vi "SC handler interface.vi"() -> ()   [LabVIEW 2011]
doc: "This VI demonstrates how to set up a GPIB board as a non system controller to simulate an instrument using the following steps:\n\nOpen a VISA session to the GPIB interface, set it as the non-system controller, and assign it a primary address. \nUse the VISA Enable Event VI to register the \"GPIB Listener\" Event; this event occurs when the GPIB interface is addressed as a listener. \nUse the VISA Wait on Event VI to wait until the GPIB interface is a listener; this means that there is data available on the bus for the interface.\nUse the VISA Read VI to read the available data, parse it, and send an appropriate response.\nCall the VISA close VI after the stop button is pressed\n\nNote: For a description of other available VISA event types, see the NI-VISA help."
uses:
  SC virtual tester states.ctl
panel:
  out "wt end hidden":u32
  out "wt start hidden":u32
  in  "sites ready hidden":string
  out "VISA close error":bool
  out "VISA error out":errorcluster
  out "VISA resource name out":refnum<visa-resource-name>
  out "VISA open error":bool
  in  "SC virtual tester states":T1
  out "H1 active":bool
  out "H2 active":bool
  out "GPIB read error":bool
  out "GPIB write error":bool
  in  "START TEST":bool
  in  "Yield variation":dbl min=-50.0 max=0.0 step=1.0
  in  "Yield set":dbl=100.0 min=0.0 max=100.0 step=1.0
  out "Wait time":dbl format="%.2f"
  in  "Test time variation":dbl=1.0 min=0.1 max=10.0 step=0.1 format="%.2f"
  out "binning string hidden":string
  out "Test time":dbl format="%.2f"
  in  "Reset Yield":bool
  out "Waiting":bool
  out "Testing":bool
  out "Duty cycle":u32(knob) caption="Duty Cycle" scale=0.0..100.0 scale format="%#.0f"
  out "Good Devices":u64
  out "Devices Tested":u64
  out "Yield":dbl format="%#.0f"
  in  "Tester talks to Sentinel Controller at":refnum<visa-resource-name>="GPIB0::1::INSTR"
  in  "Power on/off":bool=TRUE
  in  "Parallelism set":u8=8 min=1 step=1
  out "Message from tester to Sentinel Controller":string
  out "Reply from Sentinel Controller to tester":string="Response here\n"
  out "Parallelism reported by handler":u8
  out "Parallelism mismatch":bool
  in  "Test time set":dbl=1.0 min=0.1 max=10.0 step=0.1 format="%.2f"
  # "Celerint Sentinel Controller ~ Tester Simulator"
  # "%"
  # "%"
  # "%"
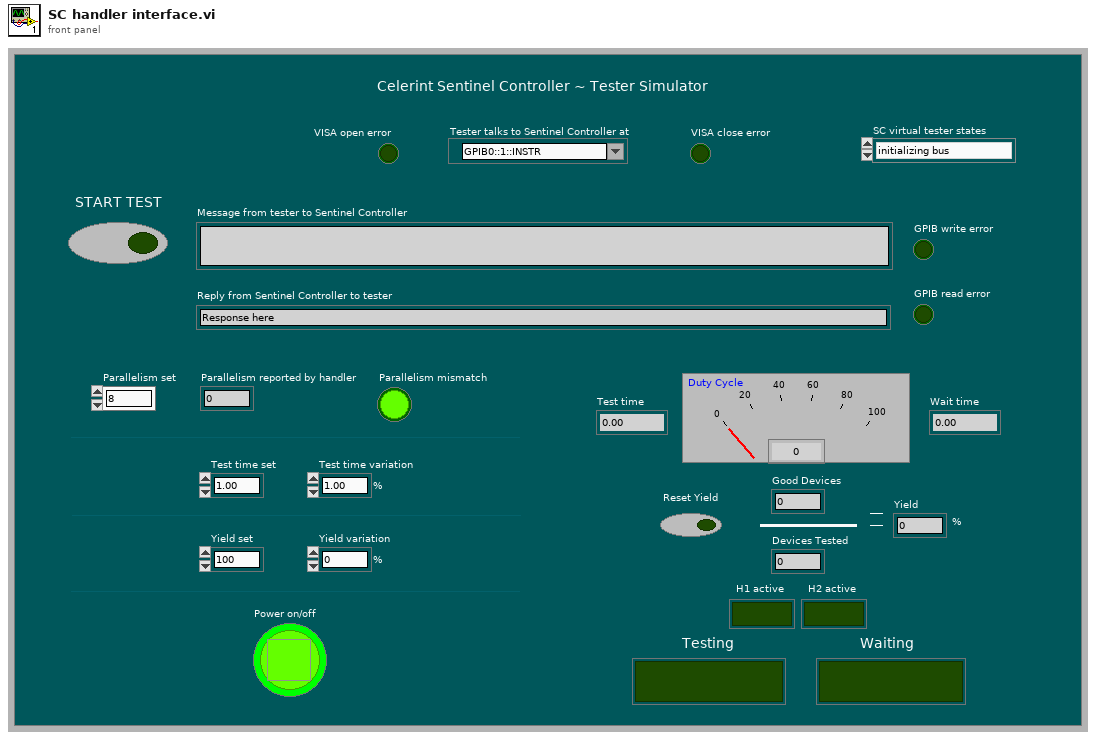
[diagram p1: front panel]
types:
  T1 = typedef "SC virtual tester states.ctl" = enum16{"initializing bus", "polling *SITES?", "sending *IDN?", "sending *HAND?", "testing", "binning", "closing bus"}
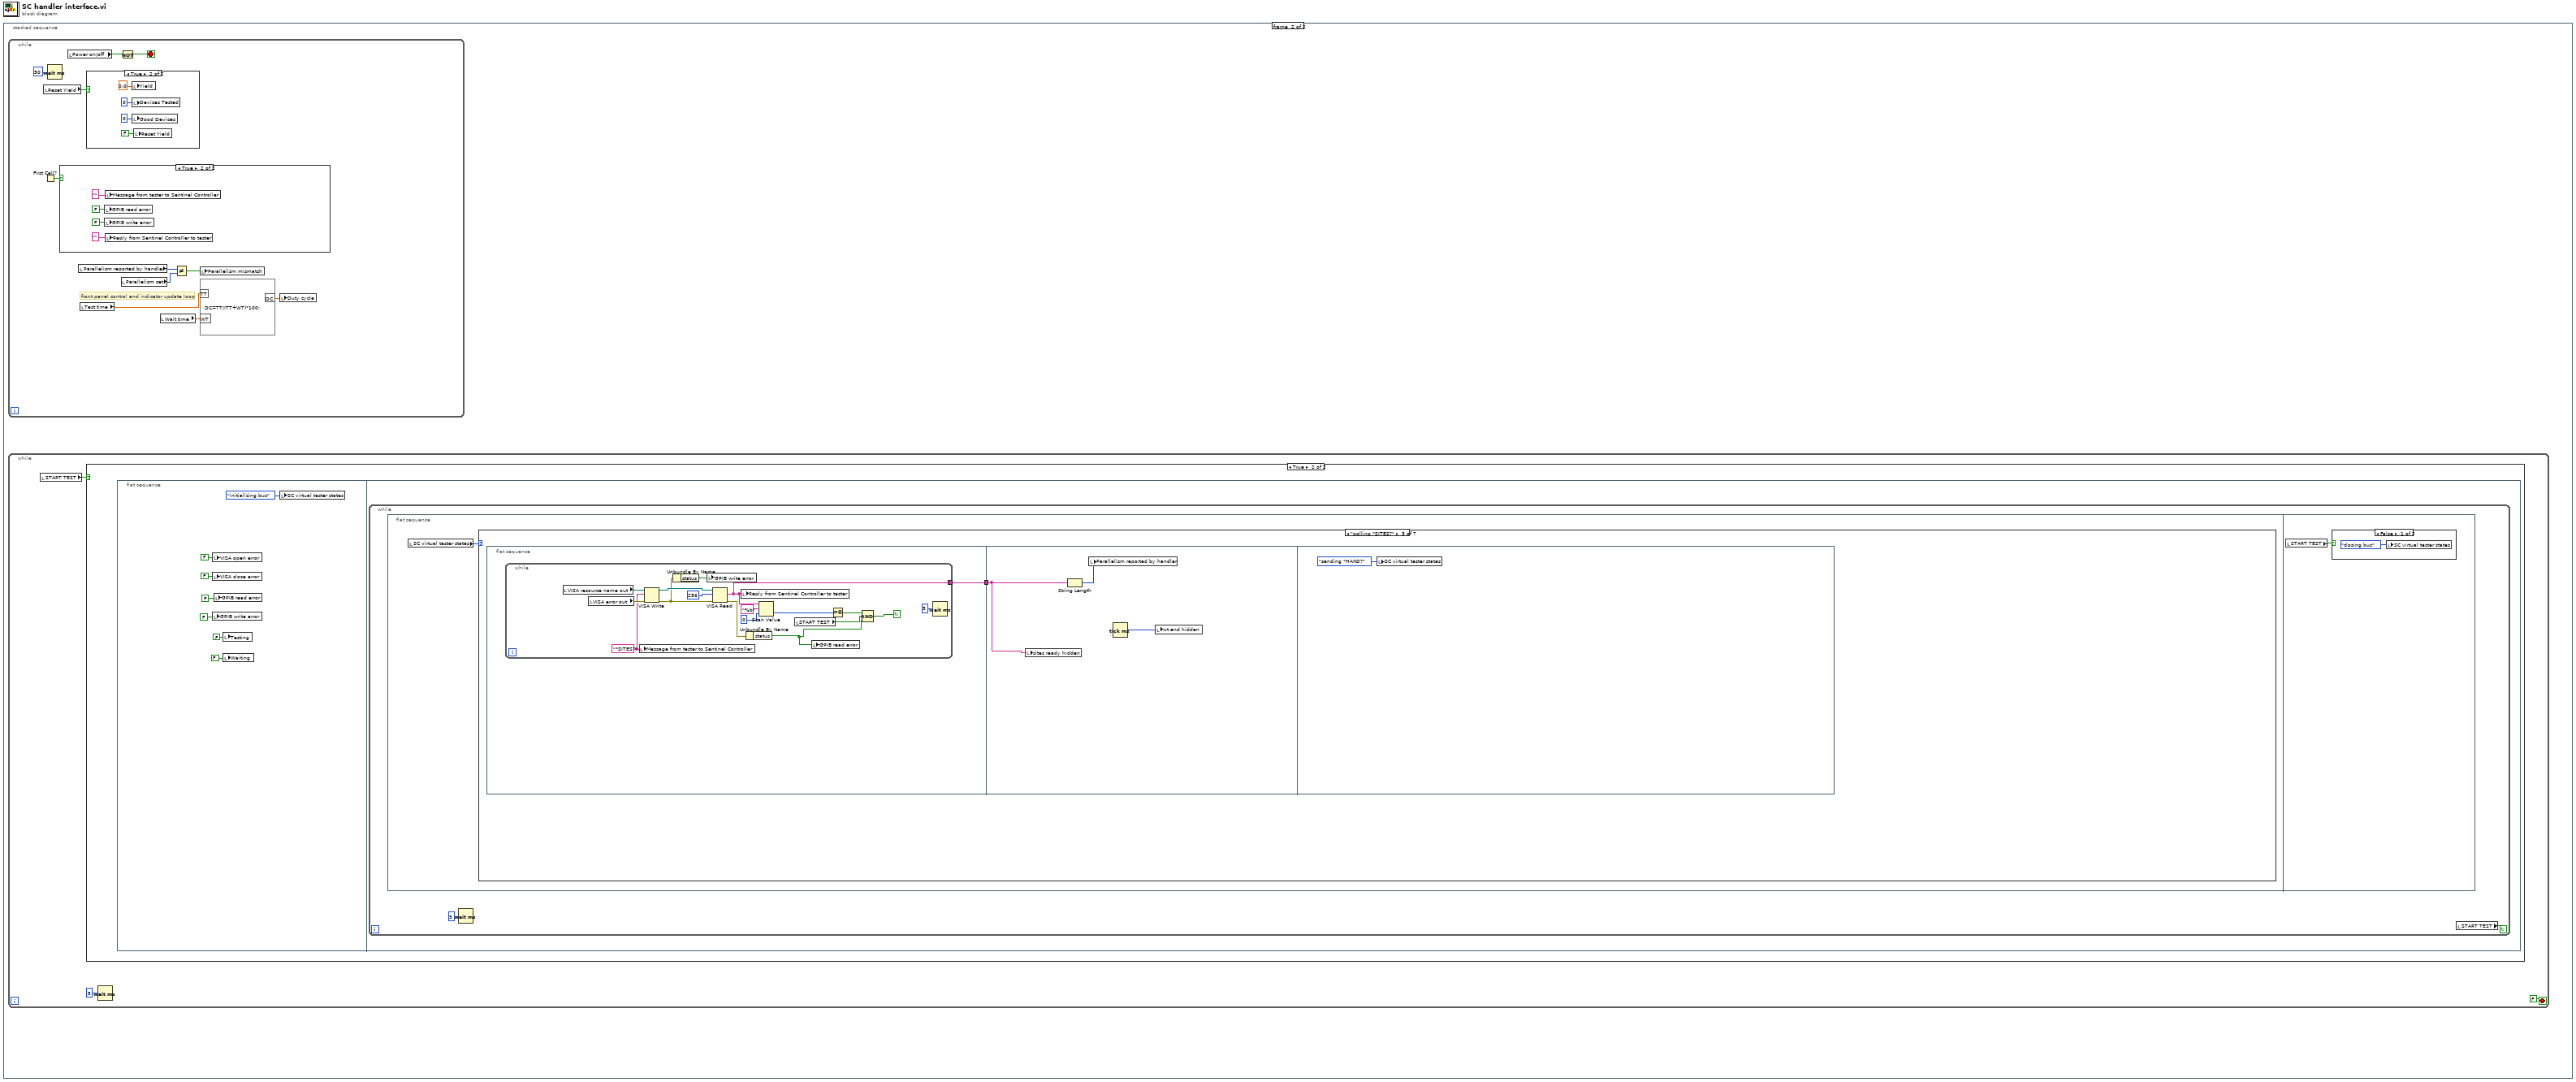
[diagram p0: block diagram]
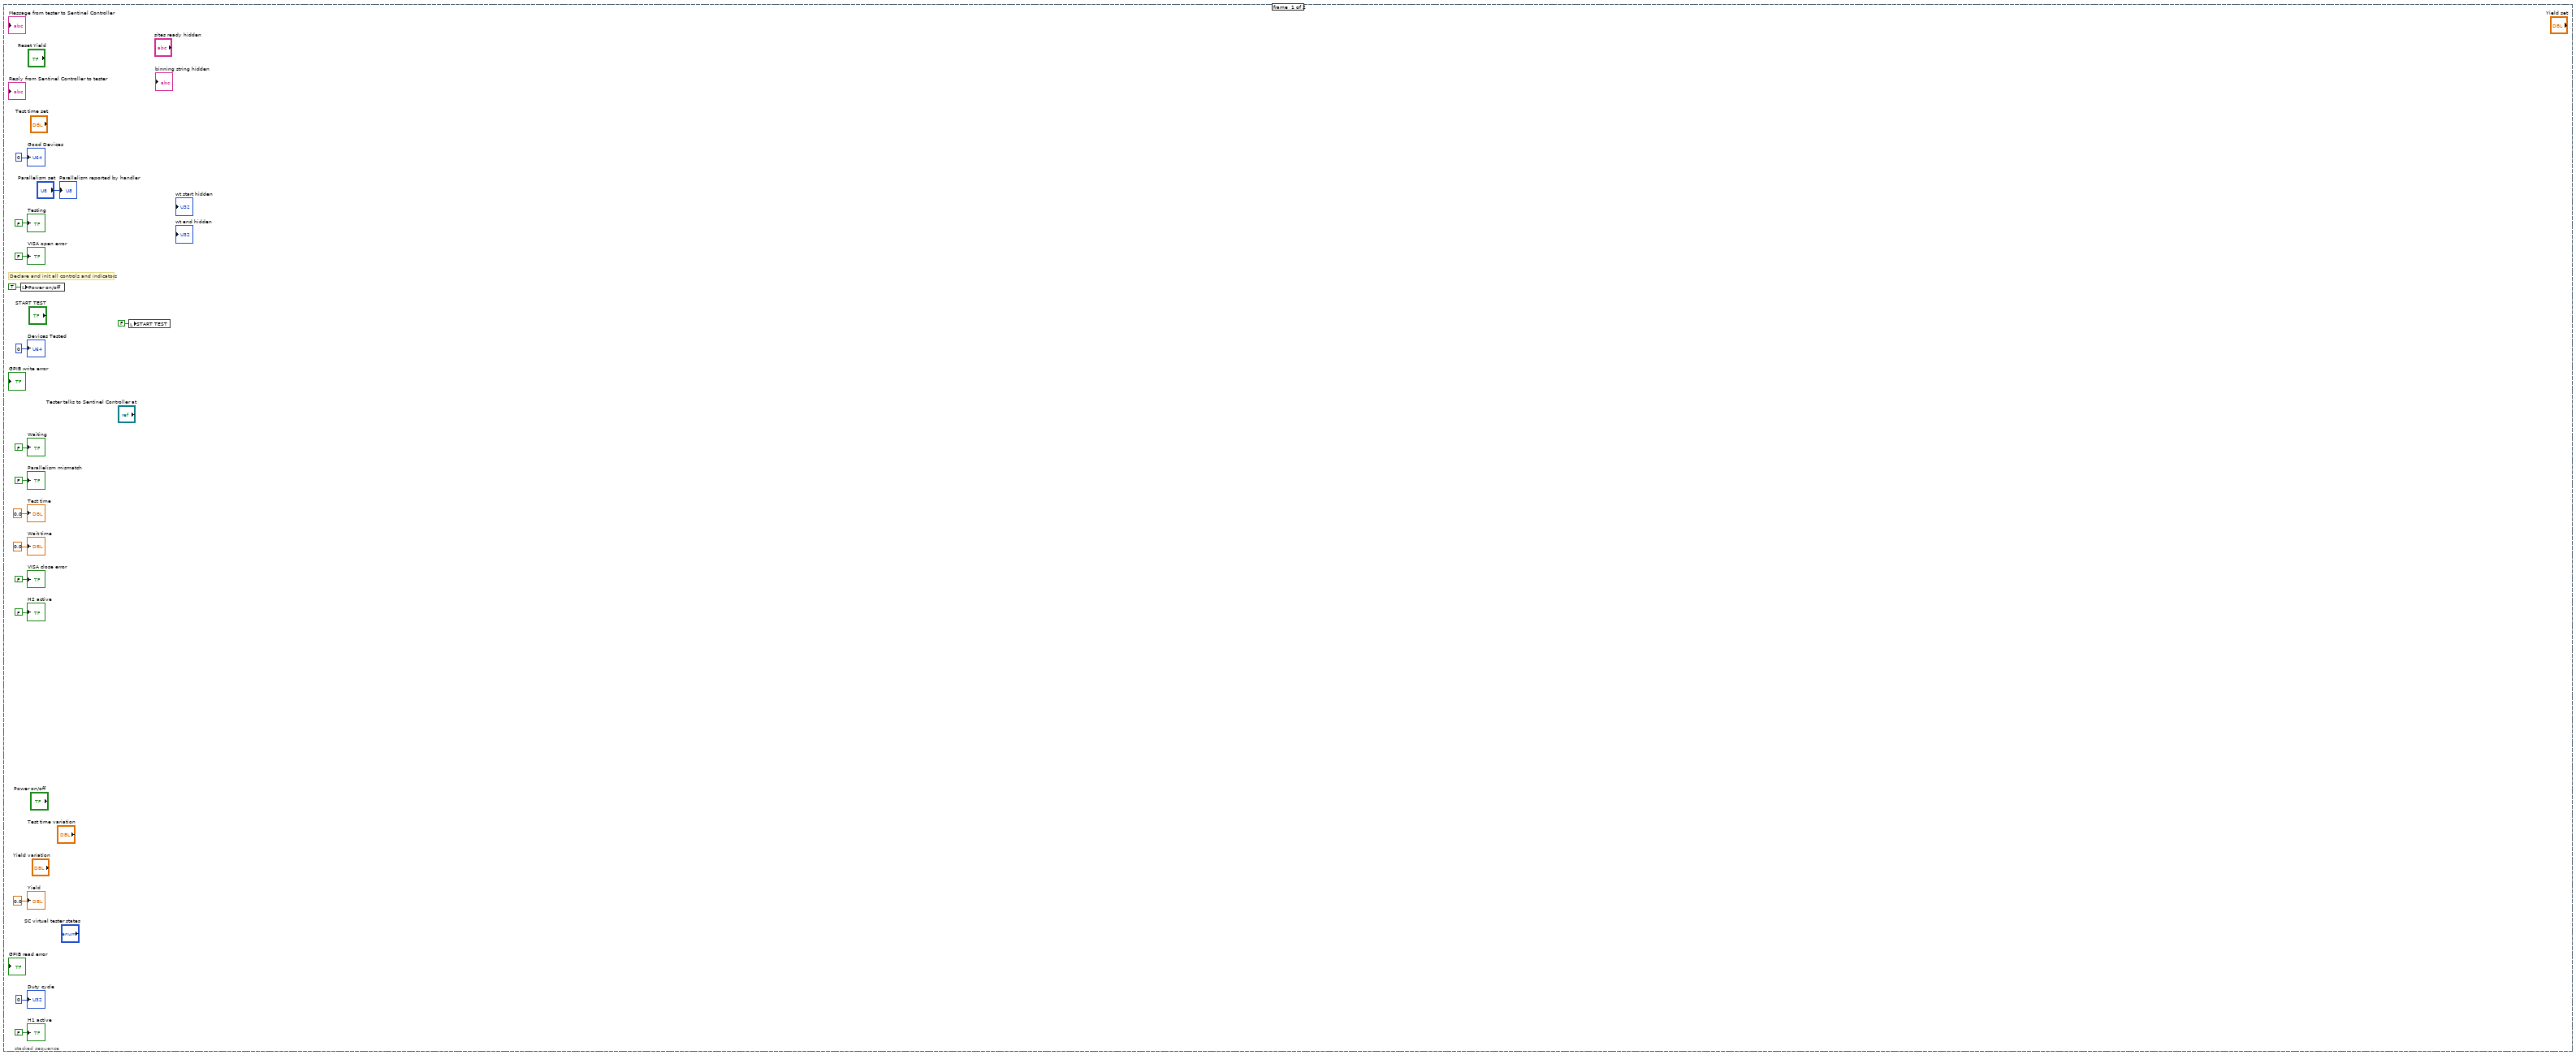
[diagram p2: hidden frame]
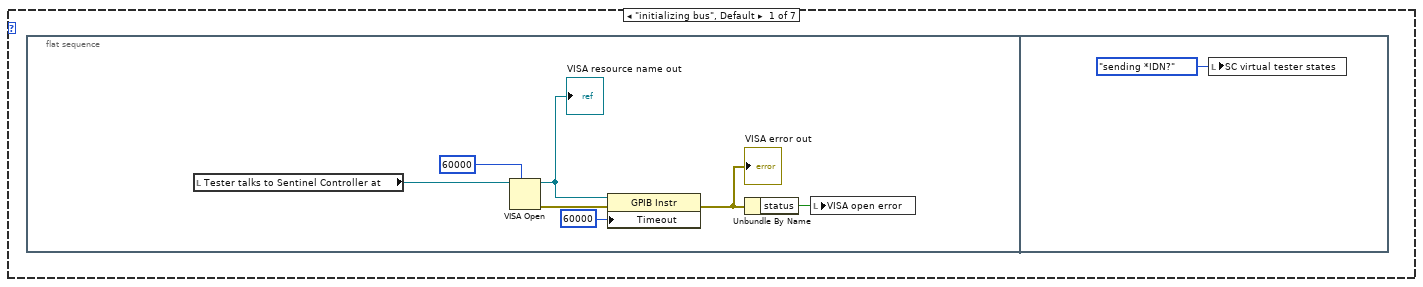
[diagram p4: hidden frame]
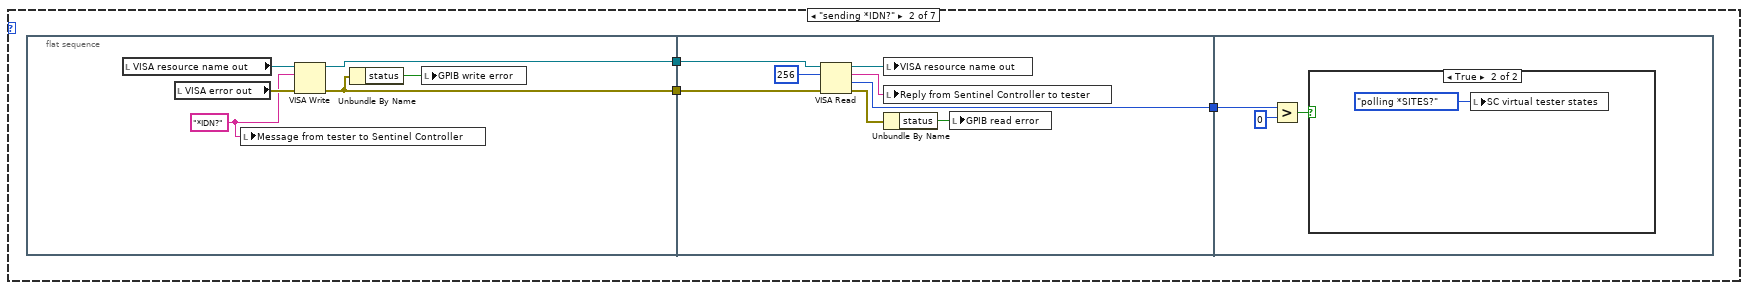
[diagram p5: hidden frame]
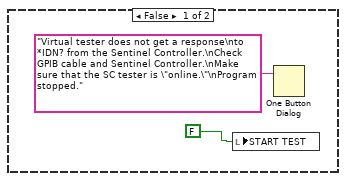
[diagram p6: hidden frame]
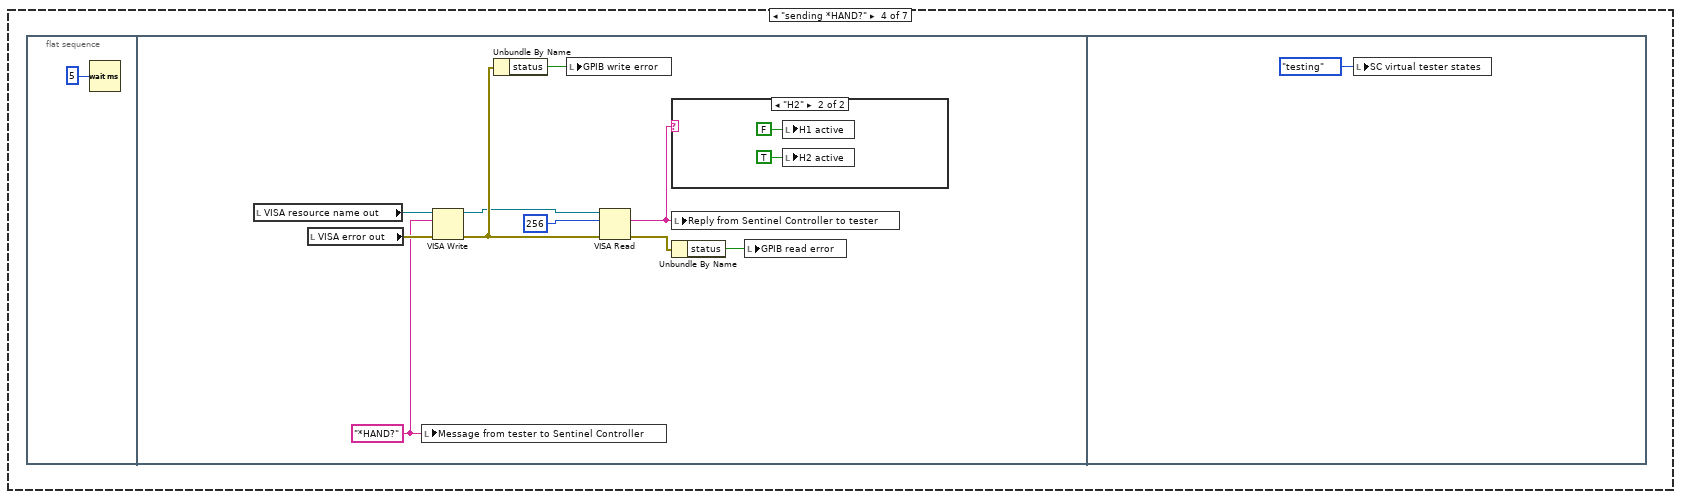
[diagram p7: hidden frame]
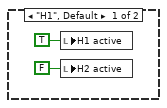
[diagram p8: hidden frame]
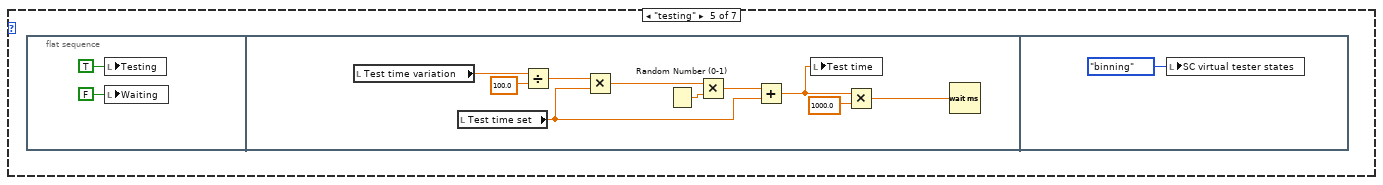
[diagram p9: hidden frame]
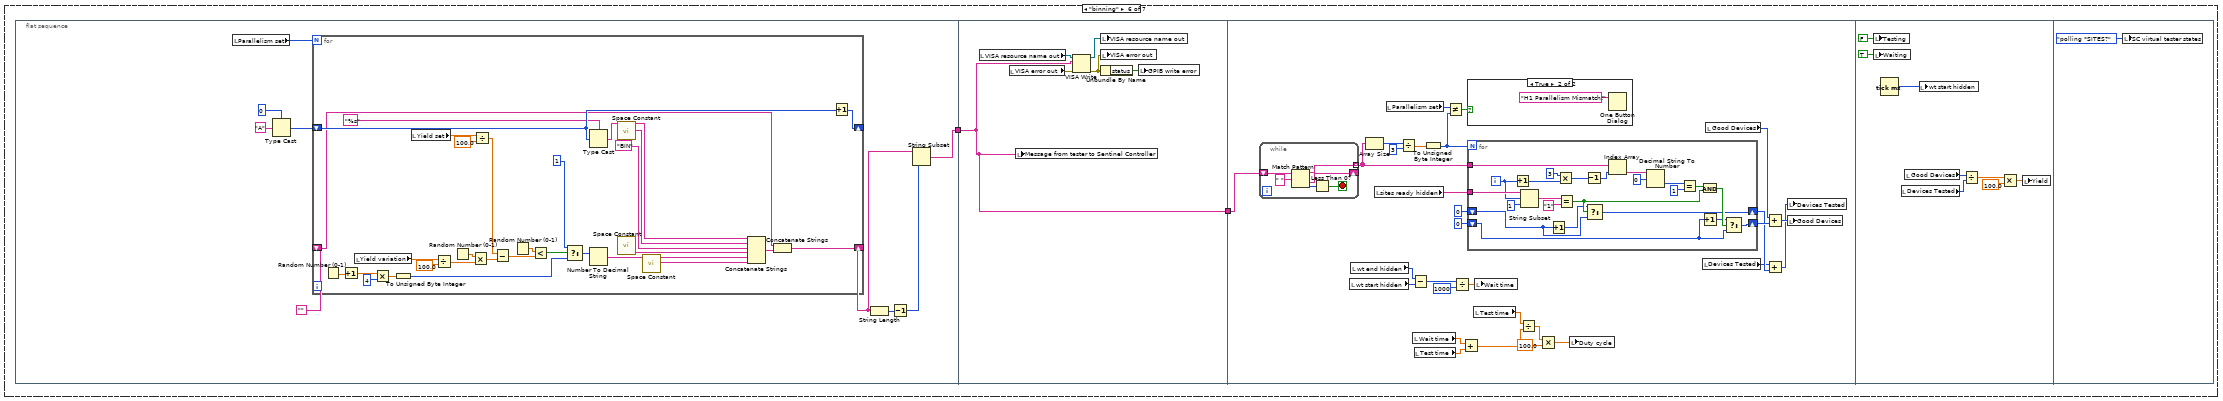
[diagram p10: hidden frame]
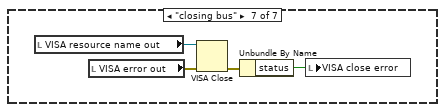
[diagram p12: hidden frame]
diagram:
  n1 = stacked-sequence {
    frame #0 {
      # "Declare and init all controls and indicators"
      n2 = local write "Power on/off"(TRUE ("Power on/off")) -> ()
      n3 = local write "START TEST"(FALSE ("START TEST")) -> ()
      "Good Devices" <- u64 0 ("Good Devices")
      "Devices Tested" <- u64 0 ("Devices Tested")
      "Yield" <- 0.0 ("Yield")
      "Waiting" <- FALSE ("Indexing")
      "Testing" <- FALSE ("Testing")
      "Duty cycle" <- u32 0 ("H1 UPH")
      "Parallelism reported by handler" <- "Parallelism set"
      "Parallelism mismatch" <- FALSE ("Parallelism mismatch")
      "Test time" <- 0.0 ("Test Time")
      "Wait time" <- 0.0 ("Wait time")
      "VISA close error" <- FALSE ("VISA close error")
      "VISA open error" <- FALSE ("VISA open error")
      "H1 active" <- FALSE ("H1 active")
      "H2 active" <- FALSE ("H2 active")
    }
    frame #1 {
      n4 = while {
        stop <- w244 stop-if-true
        # "front panel control and indicator update loop"
        n5 = local read "Reset Yield"() -> (w241:bool)
        n6 = First Call?() -> (First Call?: T/F=w237:bool)
        n7 = Wait (ms)(milliseconds to wait=u32 50) -> ()  [unwired: 1 out]
        n8 = case shown="True" w237 {
          frame False {
          }
          frame True {
            n9 = local write "GPIB read error"(FALSE ("GPIB read error")) -> ()
            n10 = local write "GPIB write error"(FALSE ("GPIB write error")) -> ()
            n11 = local write "Message from tester to Sentinel Controller"("" ("Message from tester to Sentinel Controller")) -> ()
            n12 = local write "Reply from Sentinel Controller to tester"("" ("Reply from Sentinel Controller to tester")) -> ()
          }
        }
        n13 = local read "Power on/off"() -> (w243:bool)
        n14 = local read "Parallelism reported by handler"() -> (w234:u8)
        n15 = local read "Test time"() -> (w239:dbl)
        n16 = case shown="True" w241 {
          frame False {
          }
          frame True {
            n17 = local write "Yield"(0.0 ("Yield")) -> ()
            n18 = local write "Devices Tested"(u64 0 ("Devices Tested")) -> ()
            n19 = local write "Good Devices"(u64 0 ("Good Devices")) -> ()
            n20 = local write "Reset Yield"(FALSE ("Reset Yield")) -> ()
          }
        }
        n21 = Not(x=w243) -> (.not. x?=w244:bool)
        n22 = local read "Parallelism set"() -> (w236:u8)
        n23 = local read "Wait time"() -> (w240:dbl)
        n24 = Not Equal?(x=w234, y=w236) -> (x != y?=w235:bool)
        n25 = local write "Parallelism mismatch"(w235) -> ()
        n26 = formula code="DC=TT/(TT+WT)*100;"("TT"=w239, "WT"=w240) -> ("DC"=w238:dbl)
        n27 = local write "Duty cycle"(w238) -> ()
      }
      n28 = while {
        stop <- FALSE stop-if-true
        n29 = local read "START TEST"() -> (w18:bool)
        n30 = case shown="True" w18 {
          frame False {
          }
          frame True {
            n31 = flat-sequence {
              frame #0 {
                n32 = local write "VISA open error"(FALSE ("VISA open error")) -> ()
                n33 = local write "VISA close error"(FALSE ("VISA open error")) -> ()
                n34 = local write "GPIB write error"(FALSE ("VISA open error")) -> ()
                n35 = local write "GPIB read error"(FALSE ("VISA open error")) -> ()
                n36 = local write "Testing"(FALSE ("VISA open error")) -> ()
                n37 = local write "Waiting"(FALSE ("VISA open error")) -> ()
                n38 = local write "SC virtual tester states"(SC_virtual_tester_states."initializing bus" ("SC virtual tester states")) -> ()
              }
              frame #1 {
                n39 = while {
                  stop <- w28 continue-if-true
                  n40 = flat-sequence {
                    frame #0 {
                      n41 = local read "SC virtual tester states"() -> (w29:T1)
                      n42 = case shown="\"polling *SITES?\"" w29 {
                        frame "initializing bus", Default {
                          n43 = flat-sequence {
                            frame #0 {
                              n44 = local read "Tester talks to Sentinel Controller at"() -> (w30:refnum<visa-resource-name>)
                              n45 = VISA Open(timeout (0)=u32 60000 ("VISA Open timeout (0)"), VISA resource name=w30) -> (VISA resource name=w35:refnum<visa-resource-name>, error out=w34:errorcluster)  [unwired: 3 in]
                              "VISA resource name out" <- w35
                              n46 = property class="GPIB Instr"(reference=w35, error in=w34, "Timeout"=u32 60000 ("VISA Open timeout (0)")) -> (error out=w32:errorcluster)  [unwired: 1 out]
                              "VISA error out" <- w32
                              n47 = Unbundle By Name(w32) -> ("status"=w31:bool)
                              n48 = local write "VISA open error"(w31) -> ()
                            }
                            frame #1 {
                              n49 = local write "SC virtual tester states"(SC_virtual_tester_states."sending *IDN?" ("SC virtual tester states")) -> ()
                            }
                          }
                        }
                        frame "sending *IDN?" {
                          n50 = flat-sequence {
                            tunnel: [w42] -> w40
                            tunnel: [w41] -> w39
                            tunnel: w40 -> [w54]
                            tunnel: w39 -> [w53]
                            tunnel: [w49] -> w38
                            tunnel: w38 -> [w57]
                            frame #0 {
                              w43 = "*IDN?"
                              n51 = local read "VISA resource name out"() -> (w46:refnum<visa-resource-name>)
                              n52 = local read "VISA error out"() -> (w45:errorcluster)
                              n53 = local write "Message from tester to Sentinel Controller"(w43) -> ()
                              n54 = VISA Write(VISA resource name=w46, write buffer=w43, error in (no error)=w45) -> (VISA resource name out=w42:refnum<visa-resource-name>, error out=w41:errorcluster)  [unwired: 1 out]
                              n55 = Unbundle By Name(w41) -> ("status"=w44:bool)
                              n56 = local write "GPIB write error"(w44) -> ()
                            }
                            frame #1 {
                              n57 = VISA Read(VISA resource name=w54, byte count=u32 256, error in (no error)=w53) -> (VISA resource name out=w51:refnum<visa-resource-name>, read buffer=w50:string, return count=w49:u32, error out=w47:errorcluster)
                              n58 = local write "VISA resource name out"(w51) -> ()
                              n59 = local write "Reply from Sentinel Controller to tester"(w50) -> ()
                              n60 = Unbundle By Name(w47) -> ("status"=w48:bool)
                              n61 = local write "GPIB read error"(w48) -> ()
                            }
                            frame #2 {
                              n62 = Greater?(x=w57, y=u32 0) -> (0:w55:bool)
                              n63 = case shown="True" w55 {
                                frame False {
                                n64 = local write "START TEST"(FALSE ("START")) -> ()
                                n65 = One Button Dialog(message="Virtual tester does not get a response\nto *IDN? from the Sentinel Controller.\nCheck GPIB cable and Sentinel Controller.\nMake sure that the SC tester is \"online.\"\nProgram stopped.") -> ()  [unwired: 1 in, 1 out]
                                }
                                frame True {
                                n66 = local write "SC virtual tester states"(SC_virtual_tester_states."polling *SITES?" ("SC virtual tester states")) -> ()
                                }
                              }
                            }
                          }
                        }
                        frame "polling *SITES?" {
                          n67 = flat-sequence {
                            tunnel: [w62] -> w61
                            tunnel: w61 -> [w81]
                            frame #0 {
                              n68 = while {
                                tunnel: [w64] -> w62
                                stop <- w69 continue-if-true
                                w68 = "*SITES?"
                                n69 = local read "VISA resource name out"() -> (w79:refnum<visa-resource-name>)
                                n70 = local read "VISA error out"() -> (w78:errorcluster)
                                n71 = local write "Message from tester to Sentinel Controller"(w68) -> ()
                                n72 = VISA Write(VISA resource name=w79, write buffer=w68, error in (no error)=w78) -> (VISA resource name out=w75:refnum<visa-resource-name>, error out=w66:errorcluster)  [unwired: 1 out]
                                n73 = Unbundle By Name(w66) -> ("status"=w67:bool)
                                n74 = local write "GPIB write error"(w67) -> ()
                                n75 = VISA Read(VISA resource name=w75, byte count=u32 256, error in (no error)=w66) -> (read buffer=w64:string, error out=w74:errorcluster)  [unwired: 2 out]
                                n76 = local write "Reply from Sentinel Controller to tester"(w64) -> ()
                                n77 = Unbundle By Name(w74) -> ("status"=w63:bool)
                                n78 = Scan Value(string=w64, format string="%b", default (0 dbl)=u8 0) -> (value=w71:u8)  [unwired: 1 out]
                                n79 = local read "START TEST"() -> (w65:bool)
                                n80 = local write "GPIB read error"(w63) -> ()
                                n81 = Equal To 0?(x=w71) -> (x = 0?=w70:bool)
                                n82 = Compound Arithmetic op=AND(w70, w65, w63) -> (w69:bool)
                                n83 = Wait (ms)(milliseconds to wait=u32 5) -> ()  [unwired: 1 out]
                              }
                            }
                            frame #1 {
                              n84 = local write "sites ready hidden"(w81) -> ()
                              n85 = String Length(string=w81) -> (length=w82:i32)
                              n86 = local write "Parallelism reported by handler"(w82) -> ()
                              n87 = Tick Count (ms)() -> (millisecond timer value=w80:u32)
                              n88 = local write "wt end hidden"(w80) -> ()
                            }
                            frame #2 {
                              n89 = local write "SC virtual tester states"(SC_virtual_tester_states."sending *HAND?" ("SC virtual tester states")) -> ()
                            }
                          }
                        }
                        frame "sending *HAND?" {
                          n90 = flat-sequence {
                            frame #0 {
                              n91 = Wait (ms)(milliseconds to wait=u32 5) -> ()  [unwired: 1 out]
                            }
                            frame #1 {
                              w86 = "*HAND?"
                              n92 = local read "VISA resource name out"() -> (w94:refnum<visa-resource-name>)
                              n93 = local read "VISA error out"() -> (w93:errorcluster)
                              n94 = local write "Message from tester to Sentinel Controller"(w86) -> ()
                              n95 = VISA Write(VISA resource name=w94, write buffer=w86, error in (no error)=w93) -> (VISA resource name out=w89:refnum<visa-resource-name>, error out=w90:errorcluster)  [unwired: 1 out]
                              n96 = Unbundle By Name(w90) -> ("status"=w92:bool)
                              n97 = local write "GPIB write error"(w92) -> ()
                              n98 = VISA Read(VISA resource name=w89, byte count=u32 256, error in (no error)=w90) -> (read buffer=w85:string, error out=w88:errorcluster)  [unwired: 2 out]
                              n99 = case shown="\"H2\"" w85 {
                                frame "H1", Default {
                                n100 = local write "H1 active"(TRUE ("H1 active")) -> ()
                                n101 = local write "H2 active"(FALSE ("H1 active")) -> ()
                                }
                                frame "H2" {
                                n102 = local write "H1 active"(FALSE ("H1 active")) -> ()
                                n103 = local write "H2 active"(TRUE ("H1 active")) -> ()
                                }
                              }
                              n104 = local write "Reply from Sentinel Controller to tester"(w85) -> ()
                              n105 = Unbundle By Name(w88) -> ("status"=w87:bool)
                              n106 = local write "GPIB read error"(w87) -> ()
                            }
                            frame #2 {
                              n107 = local write "SC virtual tester states"(SC_virtual_tester_states."testing" ("SC virtual tester states")) -> ()
                            }
                          }
                        }
                        frame "testing" {
                          n108 = flat-sequence {
                            frame #0 {
                              n109 = local write "Testing"(TRUE ("testing")) -> ()
                              n110 = local write "Waiting"(FALSE ("waiting")) -> ()
                            }
                            frame #1 {
                              n111 = local read "Test time variation"() -> (w108:dbl)
                              n112 = local read "Test time set"() -> (w111:dbl)
                              n113 = Divide(x=w108, y=100.0) -> (x/y=w106:dbl)
                              n114 = Multiply(x=w106, y=w111) -> (x*y=w104:dbl)
                              n115 = Random Number (0-1)() -> (number: 0 to 1=w102:dbl)
                              n116 = Multiply(x=w104, y=w102) -> (x*y=w103:dbl)
                              n117 = Add(x=w103, y=w111) -> (x+y=w110:dbl)
                              n118 = local write "Test time"(w110) -> ()
                              n119 = Multiply(x=w110, y=1000.0) -> (x*y=w109:dbl)
                              n120 = Wait (ms)(milliseconds to wait=w109) -> ()  [unwired: 1 out]
                            }
                            frame #2 {
                              n121 = local write "SC virtual tester states"(SC_virtual_tester_states."binning" ("SC virtual tester states")) -> ()
                            }
                          }
                        }
                        frame "binning" {
                          n122 = flat-sequence {
                            tunnel: [w115] -> w114
                            tunnel: w114 -> [w154]
                            tunnel: [w154] -> w113
                            tunnel: w113 -> [w180]
                            frame #0 {
                              n123 = local read "Parallelism set"() -> (w120:u8)
                              n124 = Type Cast(type=u8 0, x="A") -> (*(type *) &x=w123:u8)
                              n125 = for {
                                N: w120 -> [_]
                                shift-right: [w140] -> _
                                shift-left: w123 -> [w135]
                                shift-right: [w130] -> w116
                                shift-left: "" -> [w124]
                                n126 = Random Number (0-1)() -> (number: 0 to 1=w139:dbl)
                                n127 = Increment(x=w139) -> (x+1=w138:dbl)
                                n128 = local read "Yield variation"() -> (w144:dbl)
                                n129 = Multiply(x=w138, y=u8 4) -> (x*y=w133:dbl)
                                n130 = To Unsigned Byte Integer(number=w133) -> (unsigned 8bit integer=w136:u8)
                                n131 = local read "Yield set"() -> (w145:dbl)
                                n132 = Divide(x=w144, y=100.0) -> (x/y=w149:dbl)
                                n133 = Random Number (0-1)() -> (number: 0 to 1=w150:dbl)
                                n134 = Multiply(x=w150, y=w149) -> (x*y=w146:dbl)
                                n135 = Divide(x=w145, y=100.0) -> (x/y=w147:dbl)
                                n136 = Subtract(x=w147, y=w146) -> (x-y=w132:dbl)
                                n137 = Random Number (0-1)() -> (number: 0 to 1=w152:dbl)
                                n138 = Less?(x=w152, y=w132) -> (x < y?=w143:bool)
                                n139 = Select(t=u8 1, s=w143, f=w136) -> (s? t:f=w141:u8)
                                n140 = Type Cast(type="%s", x=w135) -> (*(type *) &x=w129:string)
                                n141 = Number To Decimal String(number=w141) -> (decimal integer string=w126:string)  [unwired: 1 in]
                                n142 = call <vilib>:"Space Constant.vi"() -> ("String"=w128:string)
                                n143 = call <vilib>:"Space Constant.vi"() -> ("String"=w127:string)
                                n144 = call <vilib>:"Space Constant.vi"() -> ("String"=w125:string)
                                n145 = Concatenate Strings(w129, w128, "BIN" ("string"), w127, w126, w125) -> (w131:string)
                                n146 = Concatenate Strings(w124, w131) -> (w130:string)
                                n147 = Increment(x=w135) -> (x+1=w140:u8)
                              }
                              n148 = String Length(string=w116) -> (length=w118:i32)
                              n149 = Decrement(x=w118) -> (x-1=w117:i32)
                              n150 = String Subset(string=w116, length (rest)=w117) -> (substring=w115:string)  [unwired: 1 in]
                            }
                            frame #1 {
                              n151 = local read "VISA resource name out"() -> (w158:refnum<visa-resource-name>)
                              n152 = local read "VISA error out"() -> (w159:errorcluster)
                              n153 = local write "Message from tester to Sentinel Controller"(w154) -> ()
                              n154 = VISA Write(VISA resource name=w158, write buffer=w154, error in (no error)=w159) -> (VISA resource name out=w155:refnum<visa-resource-name>, error out=w156:errorcluster)  [unwired: 1 out]
                              n155 = local write "VISA resource name out"(w155) -> ()
                              n156 = local write "VISA error out"(w156) -> ()
                              n157 = Unbundle By Name(w156) -> ("status"=w157:bool)
                              n158 = local write "GPIB write error"(w157) -> ()
                            }
                            frame #2 {
                              n159 = while {
                                tunnel: [w192] -> w188 mode=indexing
                                shift-right: [w193] -> _
                                shift-left: w180 -> [w195]
                                stop <- w190 stop-if-true
                                n160 = Match Pattern(string=w195, regular expression=" ") -> (before substring=w192:string, after substring=w193:string, offset past match=w191:i32)  [unwired: 2 out]
                                n161 = Less Than 0?(x=w191) -> (x < 0?=w190:bool)
                              }
                              n162 = local read "wt start hidden"() -> (w170:u32)
                              n163 = local read "wt end hidden"() -> (w171:u32)
                              n164 = Array Size(array=w188) -> (size(s)=w185:i32)
                              n165 = local read "sites ready hidden"() -> (w179:string)
                              n166 = local read "Parallelism set"() -> (w178:u8)
                              n167 = Divide(x=w185, y=3) -> (x/y=w187:dbl)
                              n168 = Subtract(x=w171, y=w170) -> (x-y=w169:u32)
                              n169 = local read "Wait time"() -> (w165:dbl)
                              n170 = local read "Test time"() -> (w164:dbl)
                              n171 = To Unsigned Byte Integer(number=w187) -> (unsigned 8bit integer=w183:u8)
                              n172 = Not Equal?(x=w178, y=w183) -> (x != y?=w184:bool)
                              n173 = Divide(x=w169, y=u32 1000) -> (x/y=w167:dbl)
                              n174 = Add(x=w165, y=w164) -> (x+y=w163:dbl)
                              n175 = case shown="True" w184 {
                                frame False {
                                }
                                frame True {
                                n176 = One Button Dialog(message="H1 Parallelism Mismatch!") -> ()  [unwired: 1 in, 1 out]
                                }
                              }
                              n177 = for {
                                N: w183 -> [_]
                                tunnel: w188 -> [w218]
                                tunnel: w179 -> [w209]
                                shift-right: [w202] -> w174
                                shift-left: 0 -> [w201]
                                shift-right: [w198] -> w175
                                shift-left: 0 -> [w196]
                                i -> [w199]
                                n178 = Increment(x=w199) -> (x+1=w217:i32)
                                n179 = String Subset(string=w209, offset (0)=w199, length (rest)=1 ("length (rest)")) -> (substring=w205:string)
                                n180 = Increment(x=w201) -> (x+1=w200:i32)
                                n181 = Multiply(x=3, y=w217) -> (x*y=w211:i32)
                                n182 = Equal?(x=w205, y="1") -> (x = y?=w203:bool)
                                n183 = Decrement(x=w211) -> (x-1=w210:i32)
                                n184 = Select(t=w200, s=w203, f=w201) -> (s? t:f=w202:i32)
                                n185 = Index Array(array=w218, index=w210) -> (element=w215:string)
                                n186 = Decimal String To Number(string=w215, offset=0) -> (number=w213:i32)  [unwired: 1 in, 1 out]
                                n187 = Equal?(x=w213, y=1) -> (x = y?=w206:bool)
                                n188 = And(x=w206, y=w203) -> (x .and. y?=w207:bool)
                                n189 = Increment(x=w196) -> (x+1=w197:i32)
                                n190 = Select(t=w197, s=w207, f=w196) -> (s? t:f=w198:i32)
                              }
                              n191 = local read "Test time"() -> (w166:dbl)
                              n192 = local write "Wait time"(w167) -> ()
                              n193 = Divide(x=w166, y=w163) -> (x/y=w162:dbl)
                              n194 = Multiply(x=w162, y=100.0) -> (x*y=w160:dbl)
                              n195 = local write "Duty cycle"(w160) -> ()
                              n196 = local read "Devices Tested"() -> (w173:u64)
                              n197 = local read "Good Devices"() -> (w176:u64)
                              n198 = Add(x=w176, y=w175) -> (x+y=w177:u64)
                              n199 = Add(x=w173, y=w174) -> (x+y=w172:u64)
                              n200 = local write "Devices Tested"(w172) -> ()
                              n201 = local write "Good Devices"(w177) -> ()
                            }
                            frame #3 {
                              n202 = local write "Testing"(FALSE ("waiting")) -> ()
                              n203 = local write "Waiting"(TRUE ("testing")) -> ()
                              n204 = Tick Count (ms)() -> (millisecond timer value=w219:u32)
                              n205 = local read "Devices Tested"() -> (w221:u64)
                              n206 = local read "Good Devices"() -> (w220:u64)
                              n207 = local write "wt start hidden"(w219) -> ()
                              n208 = Divide(x=w220, y=w221) -> (x/y=w222:dbl)
                              n209 = Multiply(x=w222, y=100.0) -> (x*y=w224:dbl)
                              n210 = local write "Yield"(w224) -> ()
                            }
                            frame #4 {
                              n211 = local write "SC virtual tester states"(SC_virtual_tester_states."polling *SITES?" ("SC virtual tester states")) -> ()
                            }
                          }
                        }
                        frame "closing bus" {
                          n212 = local read "VISA resource name out"() -> (w231:refnum<visa-resource-name>)
                          n213 = local read "VISA error out"() -> (w230:errorcluster)
                          n214 = VISA Close(VISA resource name=w231, error in (no error)=w230) -> (error out=w229:errorcluster)
                          n215 = Unbundle By Name(w229) -> ("status"=w228:bool)
                          n216 = local write "VISA close error"(w228) -> ()
                        }
                      }
                    }
                    frame #1 {
                      n217 = local read "START TEST"() -> (w232:bool)
                      n218 = case shown="False" w232 {
                        frame False {
                          n219 = local write "SC virtual tester states"(SC_virtual_tester_states."closing bus" ("SC virtual tester states")) -> ()
                        }
                        frame True {
                        }
                      }
                    }
                  }
                  n220 = Wait (ms)(milliseconds to wait=u32 5) -> ()  [unwired: 1 out]
                  n221 = local read "START TEST"() -> (w28:bool)
                }
              }
            }
          }
        }
        n222 = Wait (ms)(milliseconds to wait=u32 5) -> ()  [unwired: 1 out]
      }
    }
  }
